vi "Set Osc Channel Rangem V.vi"(8 "error in (no error)":errorcluster, 9 "maxmv":i32, 10 "minmv":i32, 11 "channel":i32) -> (0 "error out":errorcluster, 3 "function return":i32)   [LabVIEW 2021, in "vmmso.lvlib"]
doc: "DLL_API int WINAPI SetOscChannelRangemV(int channel, int minmv, int maxmv);"
uses:
  vmmso.lvlib
  vmmso.dll
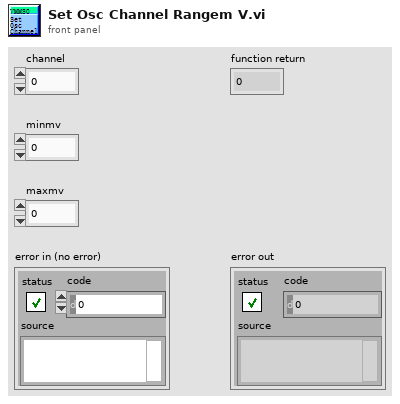
[diagram p1: front panel]
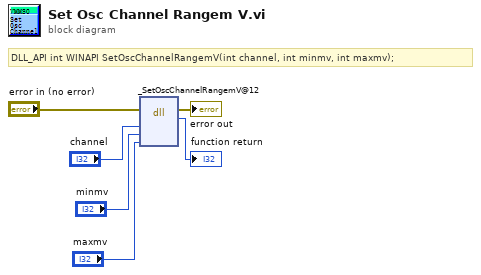
[diagram p0: block diagram]
diagram:
  # "DLL_API int WINAPI SetOscChannelRangemV(int channel, int minmv, int maxmv);"
  n1 = dll-call lib="O:/MSO/library/demo-Labview/vmmso/vmmso.*" fn="_SetOscChannelRangemV@12"(error in="error in (no error)", "channel"="channel", "minmv"="minmv", "maxmv"="maxmv") -> (error out=→"error out":errorcluster, →"function return":i32)  [unwired: 5 in, 1 out]
